vi "Enqueue with Notifier.vi"(6 "timeout in ms (-1)":i32=-1, 8 "error in":errorcluster, 9 "Data":variant, 10 "Command":string, 11 "command queue":refnum<queue>) -> (0 "error out":errorcluster, 1 "notification":variant, 4 "timed out?":bool)   [LabVIEW 2013, in "命令队列.lvlib"]
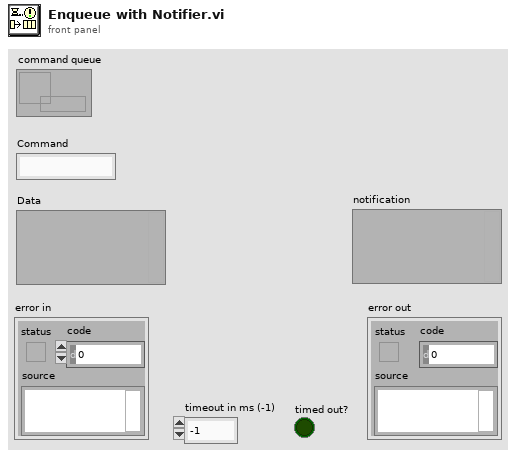
[diagram p1: front panel]
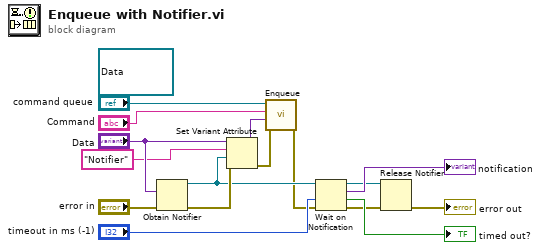
[diagram p0: block diagram]
diagram:
  (unwired) refnum<notifier> refnum ("通知器输出")
  n1 = Obtain Notifier(notification data type="Data", error in (no error)="error in") -> (notifier out=w10:refnum<notifier>, error out=w12:errorcluster)  [unwired: 2 in, 1 out]
  n2 = Set Variant Attribute(Variant="Data", name="Notifier", value=w10, error in=w12) -> (Variant out=w3:variant, error out=w4:errorcluster)  [unwired: 1 out]
  n3 = call "Enqueue.vi"("error in (no error)"=w4, "Data"=w3, "Command"="Command", "queue in"="command queue") -> ("error out"=w5:errorcluster)  [unwired: 5 in, 2 out]
  n4 = Wait on Notification(notifier=w10, timeout in ms (-1)="timeout in ms (-1)", error in (no error)=w5) -> (notifier out=w9:refnum<notifier>, notification=→"notification":variant, timed out?=→"timed out?":bool, error out=w8:errorcluster)  [unwired: 1 in]
  n5 = Release Notifier(notifier=w9, error in (no error)=w8) -> (error out=→"error out":errorcluster)  [unwired: 1 in, 2 out]
